vi "Write vRegistry.vi"(8 "error in (no error)":errorcluster, 10 "vRegistry":variant, 11 "CloneRegistration in":refnum<class "CloneRegistration.lvclass">) -> (0 "error out":errorcluster, 3 "CloneRegistration out":refnum<class "CloneRegistration.lvclass">)   [LabVIEW 2018, in "ModuleAdmin.lvlib" / "CloneRegistration.lvclass"]
uses:
  CloneRegistration.lvclass
  CloneRegistration.lvclass/CloneRegistration.ctl
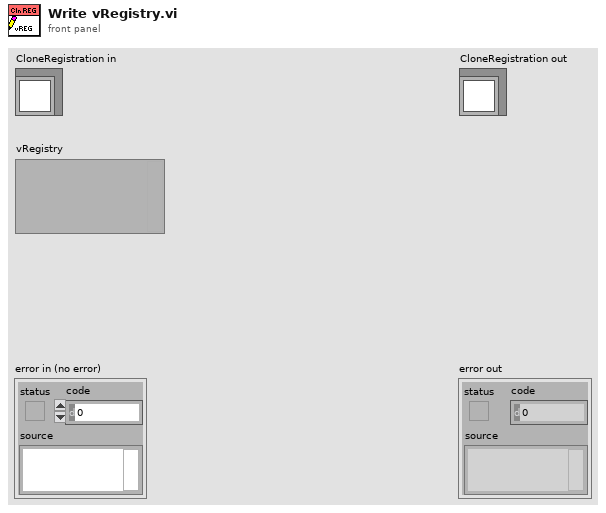
[diagram p1: front panel]
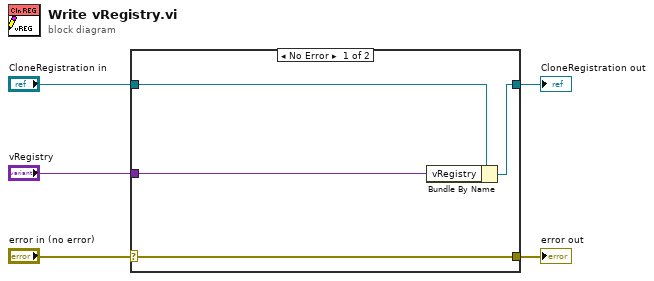
[diagram p0: block diagram]
diagram:
  n1 = case shown="No Error" "error in (no error)" {
    selector: "error in (no error)" -> [w9 w10]
    tunnel: [w9 w10] -> w4
    tunnel: [w7 w11] -> w2
    tunnel: "CloneRegistration in" -> [w8 w11]
    tunnel: "vRegistry" -> [w6 _]
    frame No Error {
      n2 = Bundle By Name(cluster=w8, "vRegistry"=w6) -> (w7:refnum<class "CloneRegistration.lvclass">)
    }
    frame Error {
    }
  }
  "error out" <- w4
  "CloneRegistration out" <- w2
